vi "Pot Calibration Finished.vi"(8 "error in (no error)":errorcluster, 10 "Pot calibratred values":cluster{"mean":dbl, "mean":dbl}, 11 "GUI Interface in":refnum<class "GUI Interface.lvclass">) -> (0 "error out":errorcluster, 3 "GUI Interface out":refnum<class "GUI Interface.lvclass">)   [LabVIEW 2020, in "GUI.lvlib" / "GUI Interface.lvclass"]
uses:
  GUI Interface.lvclass
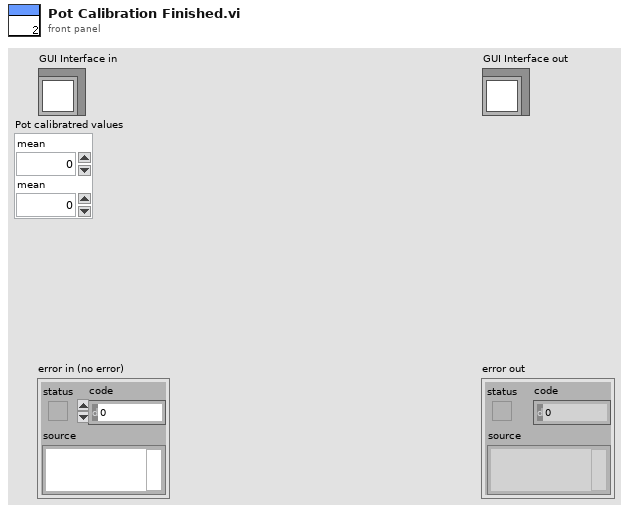
[diagram p1: front panel]
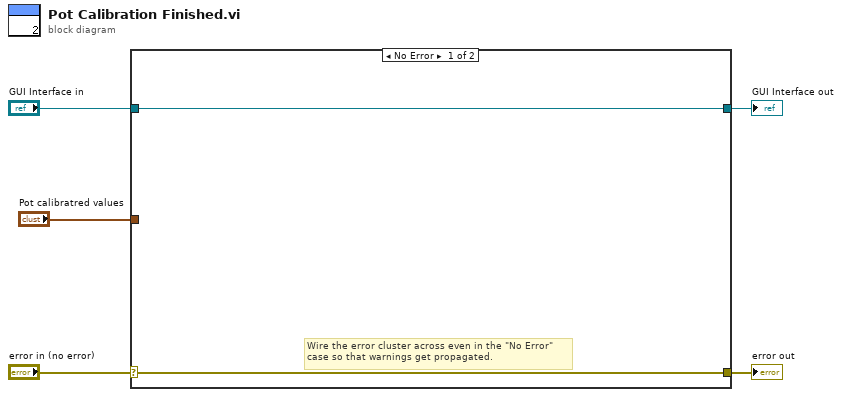
[diagram p0: block diagram]
diagram:
  n1 = case shown="No Error" "error in (no error)" {
    selector: "error in (no error)" -> [w6 w9]
    tunnel: [w6 w9] -> w4
    tunnel: [w7 w8] -> w2
    tunnel: "GUI Interface in" -> [w7 w8]
    tunnel: "Pot calibratred values" -> [_ _]
    frame No Error {
      # "Wire the error cluster across even in the \"No Error\"\ncase so that warnings get propagated."
    }
    frame Error {
    }
  }
  "error out" <- w4
  "GUI Interface out" <- w2
